vi "Run_1_of_6_Tests.vi"() -> ()   [LabVIEW 2019]
uses:
  <vilib>/Rock Robotics/WPI/ThirdParty/JAS_Junk/TrajLib/Trajectory_Library.lvlib
panel:
  out "String":string
  out "DC Motor Simulation":bool
  out "Diff Drive Kine Constraint":bool
  out "Diff Drive Voltage Constraint":bool
  out "Bang Bang Input/Output":bool
  out "Bang Bang Tolerance":bool
  out "Debounce":bool
  out "All Tests Finished":bool
  out "Diff Drive Pose Est":bool
  out "Centrip Accel Constraint":bool
  out "Controller Utility":bool
  out "Chassis Speeds":bool
  out "Cubic Spline":bool
  out "Diff Drive Kinematics":bool
  out "Angle Stats":bool
  # "FORMAL TRAJECTORY / CONTROL LIBRARY TEST PROCEDURE"
  # "FUNCTION NOT\nIMPLEMENTED"
  # "Cntrl Affine Plant Inversion"
  # "Diff Drive Odom"
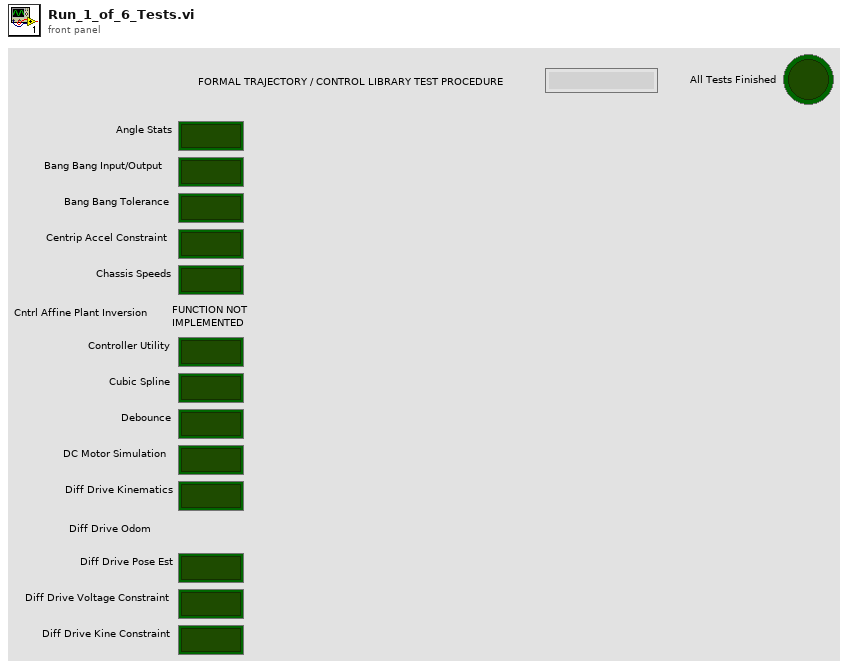
[diagram p1: front panel]
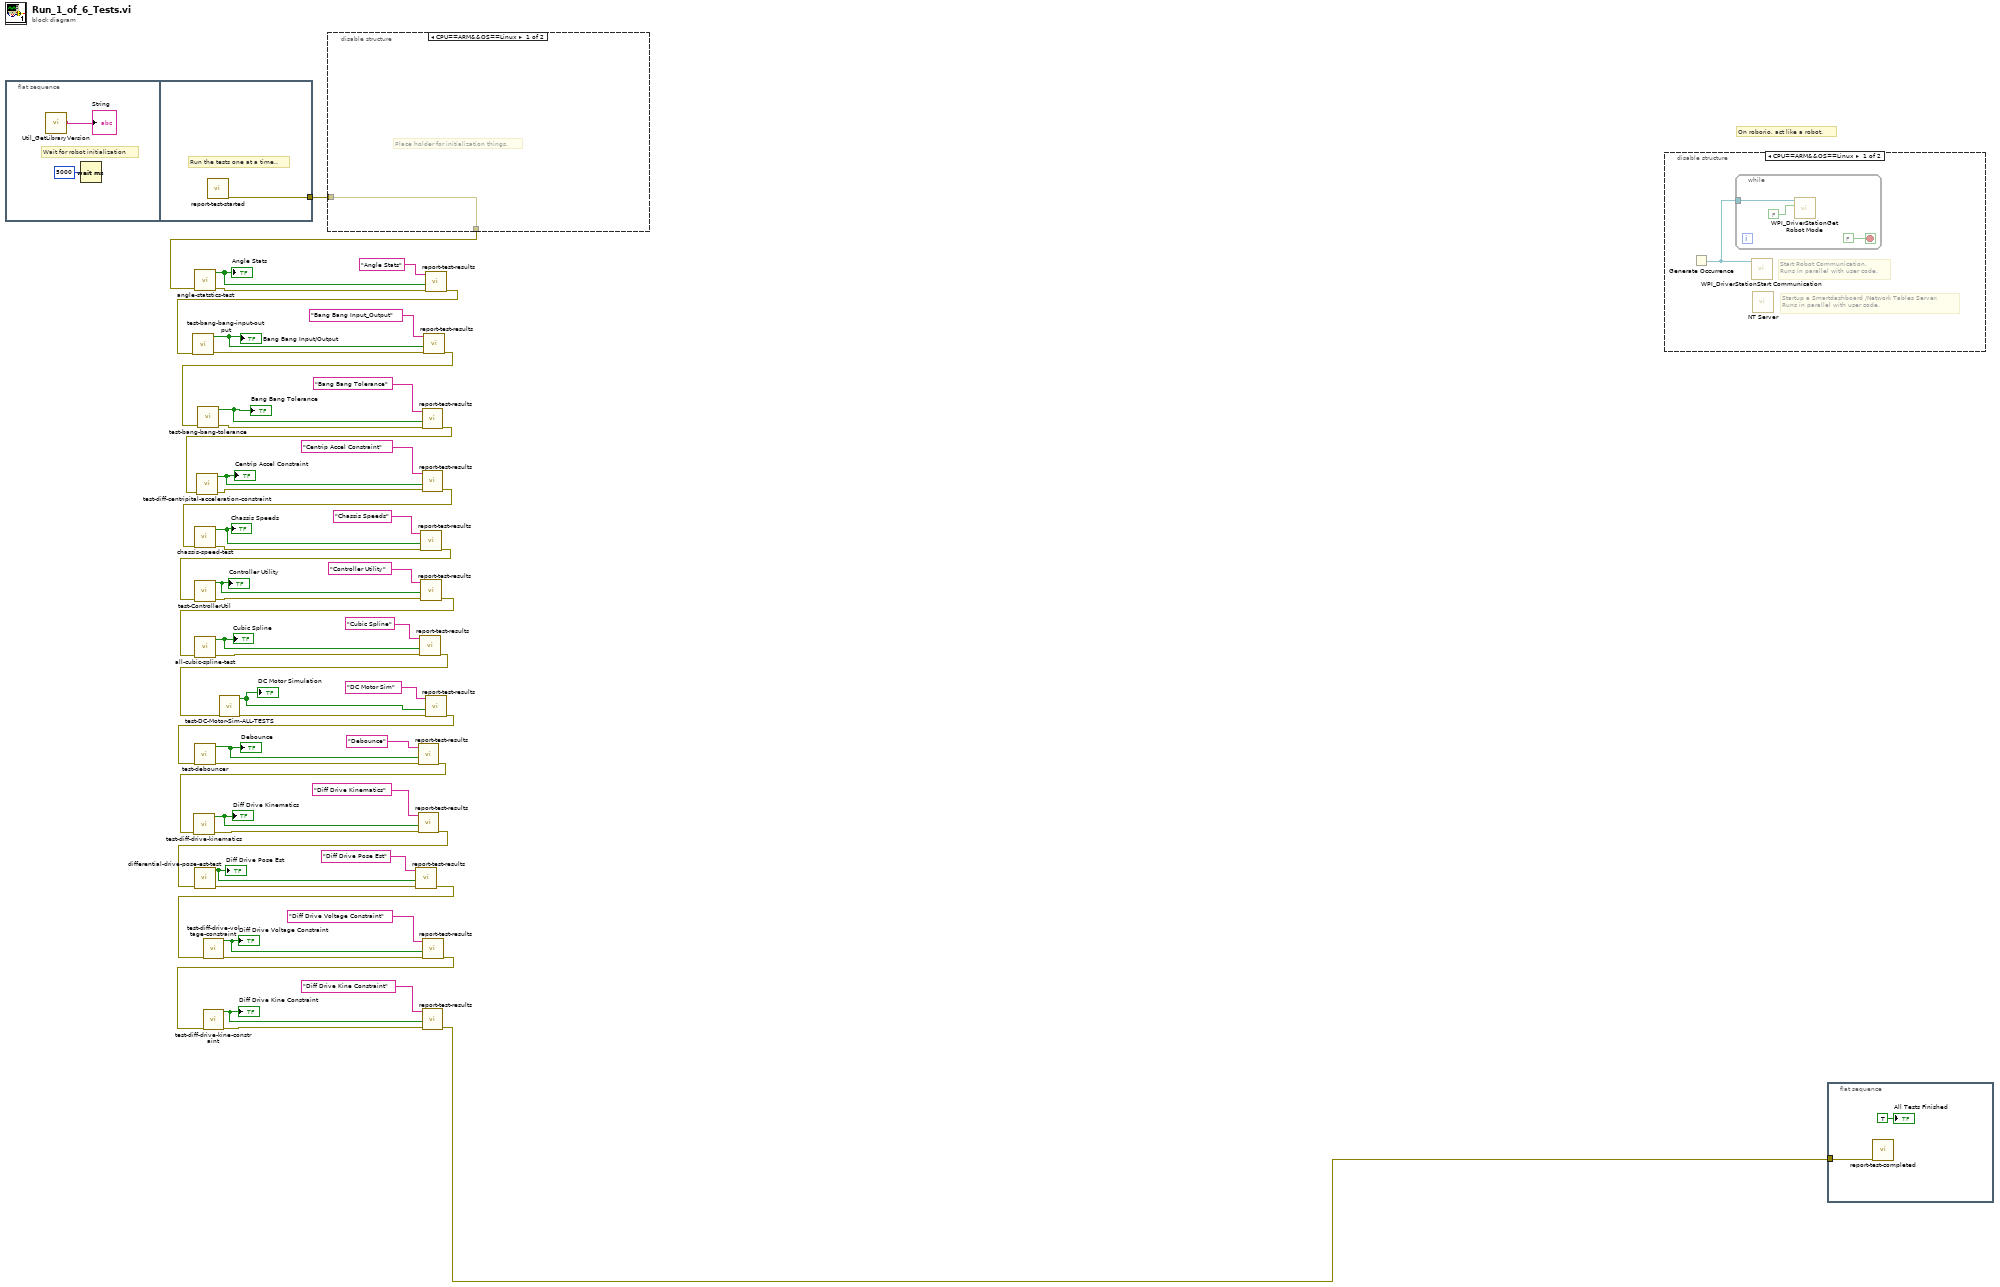
[diagram p0: block diagram]
diagram:
  # "On roborio, act like a robot."
  n1 = flat-sequence {
    tunnel: [w57] -> w16
    frame #0 {
      # "Wait for robot initialization"
      n2 = call <vilib>:"Util_GetLibraryVersion.vi"() -> ("TrajLibVersion"=→"String":string)  [unwired: 11 in]
      n3 = Wait (ms)(milliseconds to wait=u32 5000) -> ()  [unwired: 1 out]
    }
    frame #1 {
      # "Run the tests one at a time.."
      n4 = call "report-test-started.vi"() -> ("error out"=w57:errorcluster)  [unwired: 11 in]
    }
  }
  n5 = disable-structure shown="CPU==ARM&&OS==Linux" {
    disable-tunnel: w16 -> [w58 w59]
    disable-tunnel: [w58 w59] -> w15
    frame condition #0 {
      # "Place holder for initialization things."
    }
    frame condition #1 (active) {
    }
  }
  n6 = call "angle-statstics-test.vi"("error in (no error)"=w15) -> ("error out"=w34:errorcluster, "All Passed"=w54:bool)  [unwired: 9 in]
  "Angle Stats" <- w54
  n7 = call "report-test-results.vi"("error in (no error)"=w34, "TestPassed"=w54, "Test Name"="Angle Stats") -> ("error out"=w33:errorcluster)  [unwired: 8 in]
  n8 = call "test-bang-bang-input-output.vi"("error in (no error)"=w33) -> ("error out"=w32:errorcluster, "All Tests Passed"=w51:bool)  [unwired: 9 in]
  "Bang Bang Input/Output" <- w51
  n9 = call "report-test-results.vi"("error in (no error)"=w32, "TestPassed"=w51, "Test Name"="Bang Bang Input_Output") -> ("error out"=w31:errorcluster)  [unwired: 8 in]
  n10 = call "test-bang-bang-tolerance.vi"("error in (no error)"=w31) -> ("error out"=w30:errorcluster, "All Tests Passed"=w49:bool)  [unwired: 9 in]
  "Bang Bang Tolerance" <- w49
  n11 = call "report-test-results.vi"("error in (no error)"=w30, "TestPassed"=w49, "Test Name"="Bang Bang Tolerance") -> ("error out"=w29:errorcluster)  [unwired: 8 in]
  n12 = call "test-diff-centripital-acceleration-constraint.vi"("error in (no error)"=w29) -> ("error out 2"=w28:errorcluster, "Test Passed"=w47:bool)  [unwired: 9 in]
  "Centrip Accel Constraint" <- w47
  n13 = call "report-test-results.vi"("error in (no error)"=w28, "TestPassed"=w47, "Test Name"="Centrip Accel Constraint") -> ("error out"=w27:errorcluster)  [unwired: 8 in]
  n14 = call "chassis-speed-test.vi"("error in (no error)"=w27) -> ("error out"=w26:errorcluster, "Test Passed"=w45:bool)  [unwired: 9 in]
  "Chassis Speeds" <- w45
  n15 = call "report-test-results.vi"("error in (no error)"=w26, "TestPassed"=w45, "Test Name"="Chassis Speeds") -> ("error out"=w25:errorcluster)  [unwired: 8 in]
  n16 = call "test-ControllerUtil.vi"("error in (no error)"=w25) -> ("error out"=w24:errorcluster, "All Tests Passed"=w43:bool)  [unwired: 9 in]
  "Controller Utility" <- w43
  n17 = call "report-test-results.vi"("error in (no error)"=w24, "TestPassed"=w43, "Test Name"="Controller Utility") -> ("error out"=w17:errorcluster)  [unwired: 8 in]
  n18 = call "all-cubic-spline-test.vi"("error in (no error)"=w17) -> ("error out"=w23:errorcluster, "ALL TESTS PASSED"=w39:bool)  [unwired: 9 in]
  "Cubic Spline" <- w39
  n19 = call "report-test-results.vi"("error in (no error)"=w23, "TestPassed"=w39, "Test Name"="Cubic Spline") -> ("error out"=w2:errorcluster)  [unwired: 8 in]
  n20 = call "test-DC-Motor-Sim-ALL-TESTS.vi"("error in (no error)"=w2) -> ("error out"=w4:errorcluster, "All Passed"=w3:bool)  [unwired: 9 in]
  "DC Motor Simulation" <- w3
  n21 = call "report-test-results.vi"("error in (no error)"=w4, "TestPassed"=w3, "Test Name"="DC Motor Sim") -> ("error out"=w1:errorcluster)  [unwired: 8 in]
  n22 = call "test-debouncer.vi"("error in (no error)"=w1) -> ("error out"=w22:errorcluster, "ALL TESTS PASSED"=w38:bool)  [unwired: 9 in]
  "Debounce" <- w38
  n23 = call "report-test-results.vi"("error in (no error)"=w22, "TestPassed"=w38, "Test Name"="Debounce") -> ("error out"=w18:errorcluster)  [unwired: 8 in]
  n24 = call "test-diff-drive-kinematics.vi"("error in (no error)"=w18) -> ("error out"=w21:errorcluster, "All Passed"=w37:bool)  [unwired: 9 in]
  "Diff Drive Kinematics" <- w37
  n25 = call "report-test-results.vi"("error in (no error)"=w21, "TestPassed"=w37, "Test Name"="Diff Drive Kinematics") -> ("error out"=w19:errorcluster)  [unwired: 8 in]
  n26 = call "differential-drive-pose-est-test.vi"("error in (no error)"=w19) -> ("error out"=w20:errorcluster, "Test Passed"=w35:bool)  [unwired: 9 in]
  "Diff Drive Pose Est" <- w35
  n27 = call "report-test-results.vi"("error in (no error)"=w20, "TestPassed"=w35, "Test Name"="Diff Drive Pose Est") -> ("error out"=w11:errorcluster)  [unwired: 8 in]
  n28 = call "test-diff-drive-voltage-constraint.vi"("error in (no error)"=w11) -> ("error out 4"=w12:errorcluster, "Test Passed"=w13:bool)  [unwired: 9 in]
  "Diff Drive Voltage Constraint" <- w13
  n29 = call "report-test-results.vi"("error in (no error)"=w12, "TestPassed"=w13, "Test Name"="Diff Drive Voltage Constraint") -> ("error out"=w7:errorcluster)  [unwired: 8 in]
  n30 = call "test-diff-drive-kine-constraint.vi"("error in (no error)"=w7) -> ("error out 2"=w8:errorcluster, "Test Passed"=w9:bool)  [unwired: 9 in]
  "Diff Drive Kine Constraint" <- w9
  n31 = call "report-test-results.vi"("error in (no error)"=w8, "TestPassed"=w9, "Test Name"="Diff Drive Kine Constraint") -> ("error out"=w6:errorcluster)  [unwired: 8 in]
  n32 = disable-structure shown="CPU==ARM&&OS==Linux" {
    frame condition #0 {
      # "Startup a Smartdashboard /Network Tables Server.\nRuns in parallel with user code."
      # "Start Robot Communication.\nRuns in parallel with user code."
      n33 = Generate Occurrence() -> (w60:refnum<k4>)
      n34 = while {
        tunnel: w60 -> [w63]
        stop <- FALSE stop-if-true
        n35 = call <vilib>:"WPI_DriverStationGet Robot Mode.vi"("Finish"=FALSE, "DS Occurrence"=w63) -> ()  [unwired: 10 out]
      }
      n36 = call <vilib>:"WPI_DriverStationStart Communication.vi"("occurrence"=w60) -> ()  [unwired: 2 in, 9 out]
      n37 = call <vilib>:"NT Server.vi"() -> ()  [unwired: 12 in]
    }
    frame condition #1 (active) {
    }
  }
  n38 = flat-sequence {
    tunnel: w6 -> [w64]
    frame #0 {
      n39 = call "report-test-completed.vi"("error in (no error)"=w64) -> ()  [unwired: 10 in, 1 out]
      "All Tests Finished" <- TRUE ("All Tests Finished")
    }
  }
